vi "dc_fast_read_diag.vi"(8 "error in (no error)":errorcluster, 11 "DC Voltage DAQ":tag) -> (0 "error out":errorcluster, 3 "mean":dbl)   [LabVIEW 2013]
uses:
  <vilib>/DAQmx/read.llb/DAQmx Read (Analog 1D DBL 1Chan NSamp).vi
  <vilib>/Analysis/baseanly.llb/Mean (DBL).vi
  <vilib>/DAQmx/create/channels.llb/DAQmx Create Channel (AI-Voltage-Basic).vi
  <vilib>/DAQmx/configure/timing.llb/DAQmx Timing (Sample Clock).vi
  <vilib>/DAQmx/miscellaneous.llb/DAQmx Fill In Error Info.vi
  <resource>/objmgr/daqmx.rc
  <vilib>/Analysis/NI_AALBase.lvlib
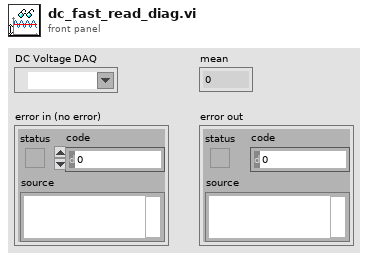
[diagram p1: front panel]
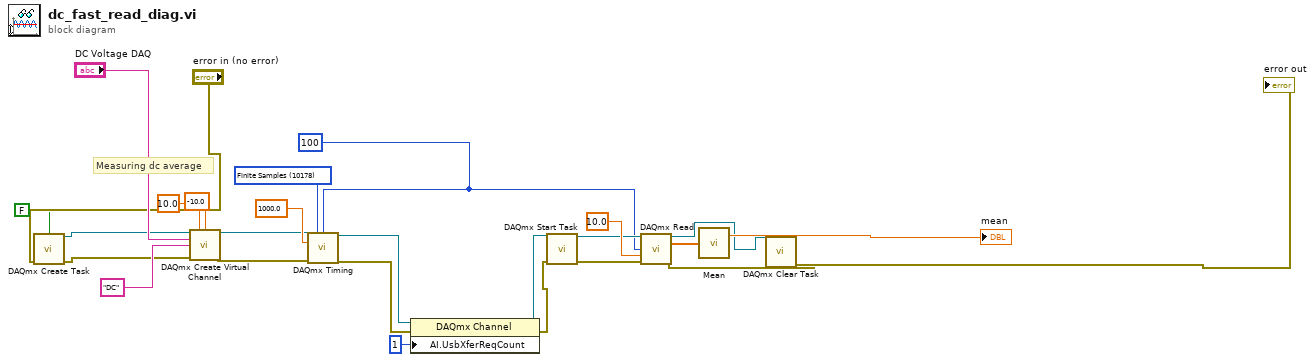
[diagram p0: block diagram]
diagram:
  w6 = 100 ("samples per channel")
  w21 = 10178 items=["Finite Samples"=10178, "Continuous Samples"=10123, "Hardware Timed Single Point"=12522] ("sample mode")
  # "Measuring dc average"
  n1 = call <vilib>:"DAQmx Create Task.vi"("auto cleanup"=FALSE, "error in"="error in (no error)") -> ("task out"=w10:refnum<k21>, "error out"=w9:errorcluster)  [unwired: 12 in]
  n2 = call-poly <vilib>:"DAQmx Create Virtual Channel.vi"("task in"=w10, "maximum value"=10.0, "minimum value"=-10.0, "physical channels"="DC Voltage DAQ", "name to assign"="DC", "error in"=w9) -> ("task out"=w15:refnum<k21>, "error out"=w17:errorcluster)  [unwired: 8 in]
  n3 = call-poly <vilib>:"DAQmx Timing.vi"("task/channels in"=w15, "sample mode"=w21, "samples per channel"=w6, "rate"=1000.0, "error in"=w17) -> ("task out"=w2:refnum<k21>, "error out"=w4:errorcluster)  [unwired: 9 in]
  n4 = property class="DAQmx Channel"(reference=w2, error in=w4, "AI.UsbXferReqCount"=u32 1) -> (reference out=w1:refnum<k21>, error out=w3:errorcluster)
  n5 = call <vilib>:"DAQmx Start Task.vi"("task/channels in"=w1, "error in"=w3) -> ("task out"=w18:refnum<k21>, "error out"=w19:errorcluster)  [unwired: 12 in]
  n6 = call-poly <vilib>:"DAQmx Read.vi"("task/channels in"=w18, "number of samples per channel"=w6, "timeout"=10.0, "error in"=w19) -> ("task out"=w24:refnum<k21>, "data"=w22:dbl[], "error out"=w23:errorcluster)  [unwired: 9 in]
  n7 = call-poly <vilib>:"Mean.vi"("X"=w22) -> ("mean"=→"mean":dbl)  [unwired: 1 out]
  n8 = call <vilib>:"DAQmx Clear Task.vi"("task in"=w24, "error in"=w23) -> ("error out"=→"error out":errorcluster)  [unwired: 13 in]
